vi "Get_Connect_Status.vi"(5 "Device Number":T1, 7 "Update":bool, 11 "Connected":bool) -> (3 "Connected":bool)   [LabVIEW 2025]
uses:
  _TypeDefs/FRIC_navX_DeviceNumbersTypeDef.ctl
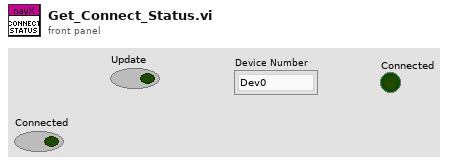
[diagram p1: front panel]
types:
  T1 = typedef "FRIC_navX_DeviceNumbersTypeDef.ctl" = enum16{"Dev0", "Dev1", "Dev2", "Dev3"}
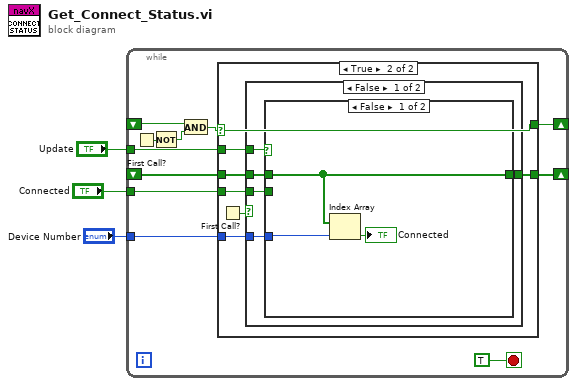
[diagram p0: block diagram]
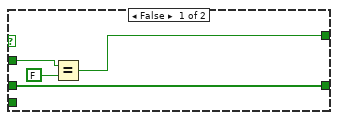
[diagram p2: hidden frame]
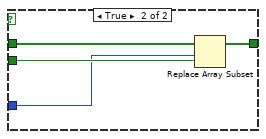
[diagram p3: hidden frame]
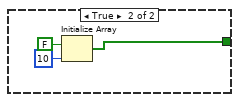
[diagram p4: hidden frame]
diagram:
  n1 = while {
    tunnel: "Update" -> [w13]
    shift-right: [w10] -> _
    shift-left: _ -> [w12]
    tunnel: "Connected" -> [w11]
    tunnel: "Device Number" -> [w9]
    shift-right: [w4] -> _
    shift-left: _ -> [w6]
    stop <- TRUE stop-if-true
    n2 = First Call?() -> (First Call?: T/F=w7:bool)
    n3 = Not(x=w7) -> (.not. x?=w8:bool)
    n4 = And(x=w6, y=w8) -> (x .and. y?=w5:bool)
    n5 = case shown="True" w5 {
      selector: w5 -> [_ w19]
      tunnel: w13 -> [w16 w25]
      tunnel: w12 -> [w18 w24]
      tunnel: w11 -> [_ w23]
      tunnel: [w18 w22] -> w10
      tunnel: w9 -> [_ w21]
      tunnel: [w15 w19] -> w4
      frame False {
        n6 = Equal?(x=w16, y=FALSE) -> (x = y?=w15:bool)
      }
      frame True {
        n7 = First Call?() -> (First Call?: T/F=w20:bool)
        n8 = case shown="False" w20 {
          tunnel: w25 -> [w30 _]
          tunnel: w24 -> [w29 _]
          tunnel: w23 -> [w28 _]
          tunnel: [w27 w38] -> w22
          tunnel: w21 -> [w26 _]
          frame False {
            n9 = case shown="False" w30 {
              tunnel: w29 -> [w32 w37]
              tunnel: w28 -> [_ w35]
              tunnel: [w32 w36] -> w27
              tunnel: w26 -> [w31 w34]
              frame False {
                n10 = Index Array(array=w32, index=w31) -> (element=→"Connected":bool)
              }
              frame True {
                n11 = Replace Array Subset(array=w37, new element=w35, index=w34) -> (w36:bool[])
              }
            }
          }
          frame True {
            n12 = Initialize Array(FALSE ("Connected"), 10 ("dimension size")) -> (w38:bool[])
          }
        }
      }
    }
  }
